vi "Read Limit(String Array).vi"(7 "Test":string, 8 "error in (no error)":errorcluster) -> (0 "error out":errorcluster, 2 "LowLimit":string[](array[string]), 3 "HighLimit":string[](array[string]))   [LabVIEW 2019, in "Unit Test Engine Tools.lvlib"]
uses:
  Unit Test Engine Tools.lvlib
  LVUT Global 1.vi
  <vilib>/Utility/file.llb/Read Delimited Spreadsheet (string).vi
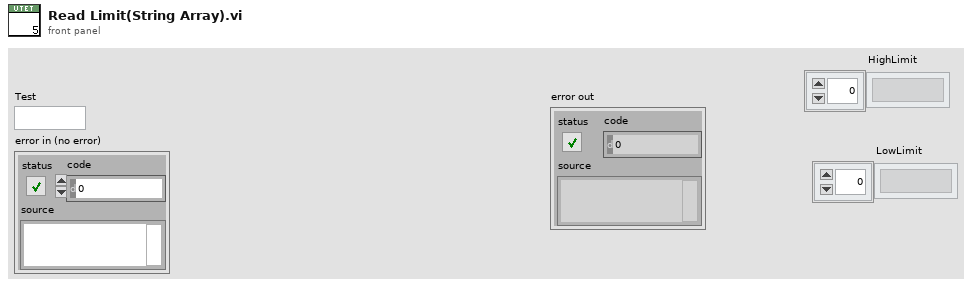
[diagram p1: front panel]
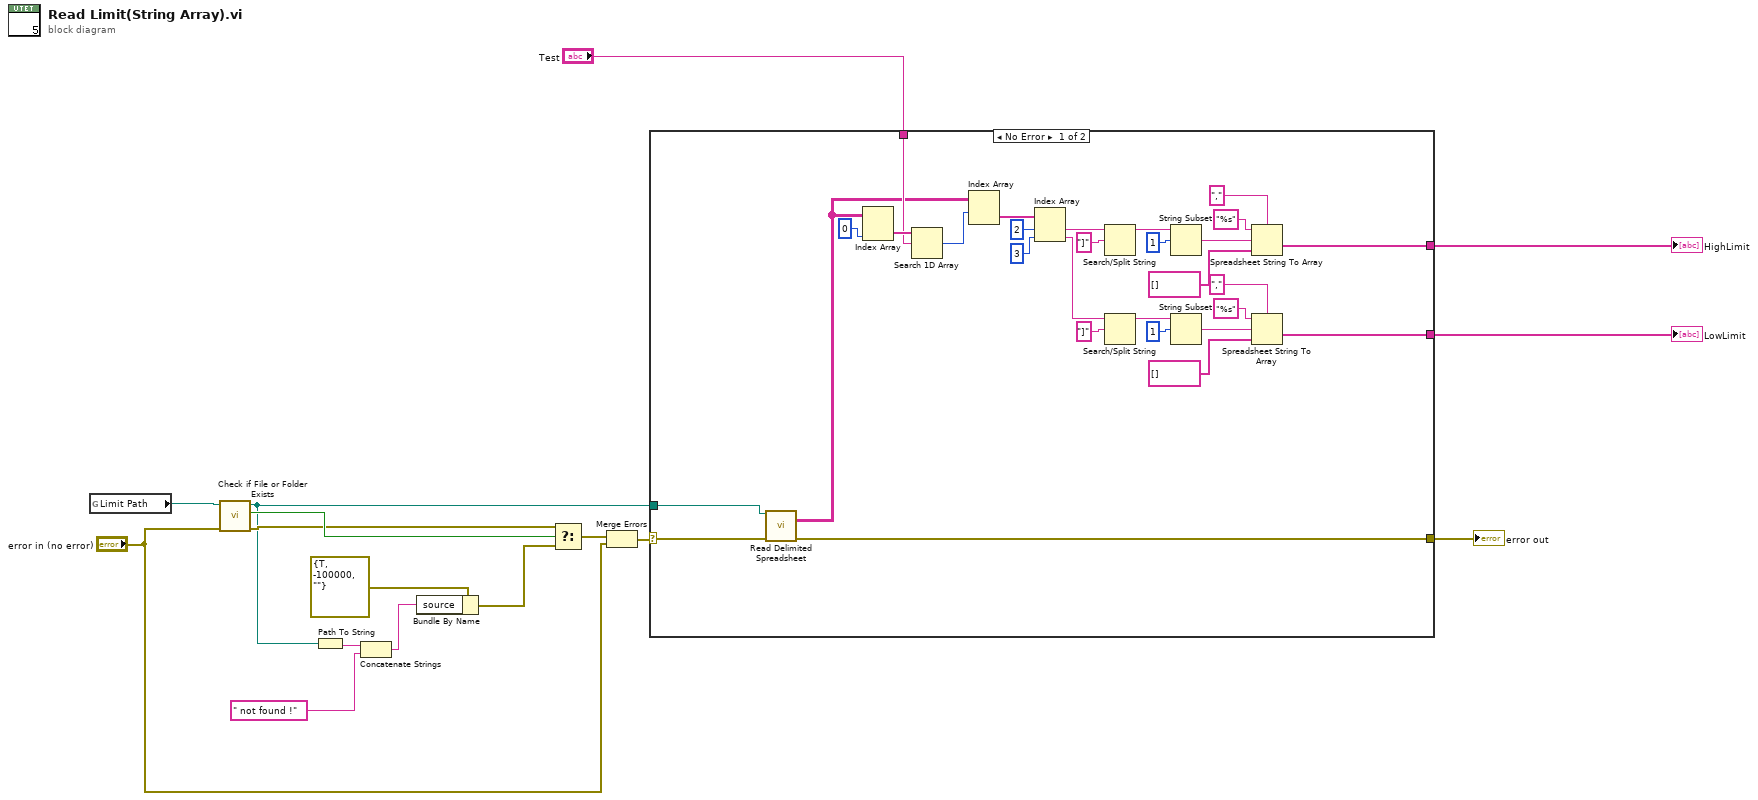
[diagram p0: block diagram]
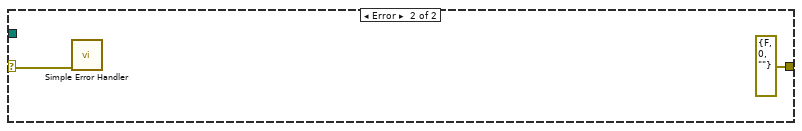
[diagram p2: hidden frame]
diagram:
  n1 = global read "LVUT Global 1.vi" "Limit Path"() -> (w10:path)
  n2 = call <vilib>:"Check if File or Folder Exists.vi"("error in (no error)"="error in (no error)", "path"=w10) -> ("error out"=w8:errorcluster, "file or folder exists?"=w9:bool, "dup path"=w2:path)  [unwired: 7 in]
  n3 = Path To String(path=w2) -> (string=w12:string)
  n4 = Concatenate Strings(w12, " not found !" ("string")) -> (w5:string)
  n5 = Bundle By Name(cluster=errorcluster {"status"=TRUE, "code"=-100000, "source"=""} ("f"), "source"=w5) -> (w6:errorcluster)
  n6 = Select(t=w8, s=w9, f=w6) -> (s? t:f=w4:errorcluster)
  n7 = Merge Errors(w4, "error in (no error)") -> (w3:errorcluster)
  n8 = case shown="No Error" w3 {
    selector: w3 -> [w19 w47]
    tunnel: "Test" -> [w43 _]
    tunnel: [w21 _] -> w15
    tunnel: [w20 _] -> w14
    tunnel: [w18 errorcluster {"status"=FALSE, "code"=0, "source"=""} ("error out")] -> w13
    tunnel: w2 -> [w17 _]
    frame No Error {
      n9 = call-poly <vilib>:"Read Delimited Spreadsheet.vi"("file path (dialog if empty)"=w17, "error in (no error)"=w19) -> ("all rows"=w42:string[][], "error out"=w18:errorcluster)  [unwired: 8 in, 4 out]
      n10 = Index Array(array=w42, index (col)=0 ("disabled index (col)")) -> (element=w44:string[])  [unwired: 1 in]
      n11 = Search 1D Array(1D array=w44, element=w43) -> (index of element=w41:i32)  [unwired: 1 in]
      n12 = Index Array(array=w42, index (row)=w41) -> (element=w40:string[])  [unwired: 1 in]
      n13 = Index Array(array=w40, index #1=2 ("index"), index #2=3 ("index")) -> (element #1=w24:string, element #2=w23:string)
      n14 = Search/Split String(string=w24, search string/char (-)="]" ("regular expression")) -> (substring before match=w36:string)  [unwired: 1 in, 2 out]
      n15 = Search/Split String(string=w23, search string/char (-)="]" ("regular expression")) -> (substring before match=w26:string)  [unwired: 1 in, 2 out]
      n16 = String Subset(string=w36, offset (0)=1) -> (substring=w37:string)  [unwired: 1 in]
      n17 = String Subset(string=w26, offset (0)=1) -> (substring=w25:string)  [unwired: 1 in]
      n18 = Spreadsheet String To Array(delimiter (Tab)=",", format string="%s", spreadsheet string=w37, array type (2D Dbl)=string[] []) -> (array=w21:string[])
      n19 = Spreadsheet String To Array(delimiter (Tab)=",", format string="%s", spreadsheet string=w25, array type (2D Dbl)=string[] []) -> (array=w20:string[])
    }
    frame Error {
      n20 = call <vilib>:"Simple Error Handler.vi"("error in (no error)"=w47) -> ()  [unwired: 4 in, 5 out]
    }
  }
  "error out" <- w13
  "HighLimit" <- w15
  "LowLimit" <- w14
